vi "Obtain Queue.vi"(8 "error in (no error)":errorcluster, 10 "Queue Name":string) -> (0 "error out":errorcluster, 3 "queue out":refnum<queue>)   [LabVIEW 2019, in "Status.lvlib"]
doc: "Function to enqueue a Message in a Queue of other Module."
uses:
  Status.lvlib
  Queue Type.ctl
  State Name.ctl
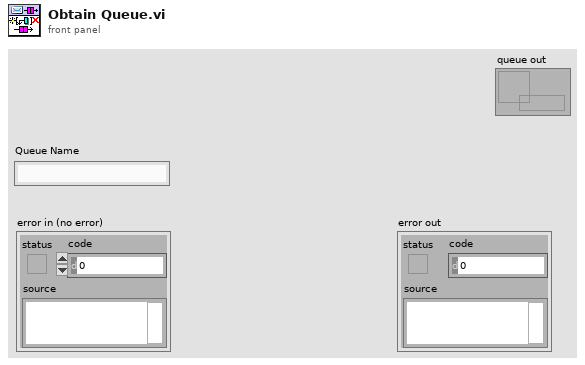
[diagram p1: front panel]
types:
  T1 = typedef "Status.lvlib/Queue Type.ctl" = cluster{"Custom State Name":string, "Defined State Name":T2, "Call Chain":string[], "Message Data":variant}
  T2 = typedef "Status.lvlib/State Name.ctl" = enum16{"Initialize", "Update Progress Bar", "Update Status Bar", "Set Cursor Busy", "Unset Cursor Busy", "Error", "Default", "Exit"}
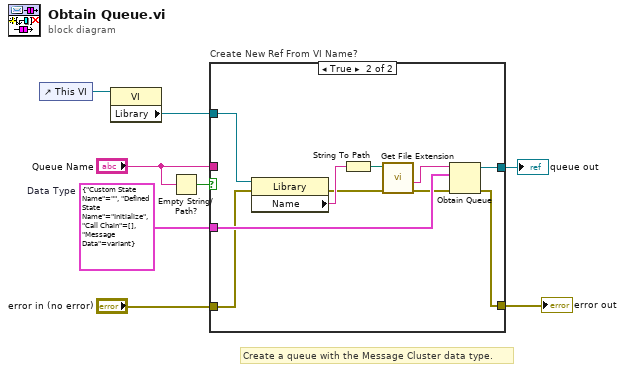
[diagram p0: block diagram]
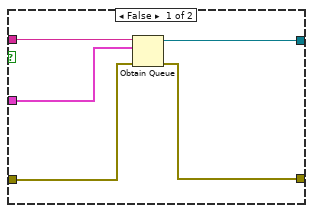
[diagram p2: hidden frame]
diagram:
  w6 = T1 {"Custom State Name"="", "Defined State Name"=enum."Initialize", "Call Chain"=[], "Message Data"=variant}  # Data Type
  # "Create a queue with the Message Cluster data type."
  n1 = control-ref of="This VI"() -> (w2:refnum<vi>)
  n2 = property class="VI"(reference=w2) -> ("Library"=w1:refnum<vi>)  [unwired: 1 in, 2 out]
  n3 = Empty String/Path?(string/path="Queue Name") -> (empty?=w8:bool)
  n4 = case "Create New Ref From VI Name?" shown="True" w8 {
    tunnel: "error in (no error)" -> [w13 w16]
    tunnel: [w12 w23] -> w5
    tunnel: [w11 w22] -> w3
    tunnel: "Queue Name" -> [w10 _]
    tunnel: w6 -> [w9 w21]
    tunnel: w1 -> [_ w20]
    frame False {
      n5 = Obtain Queue(name (unnamed)=w10, element data type=w9, error in (no error)=w13) -> (queue out=w11:refnum<queue>, error out=w12:errorcluster)  [unwired: 2 in, 1 out]
    }
    frame True {
      n6 = property class="Library"(reference=w20, error in=w16) -> (error out=w15:errorcluster, "Name"=w18:string)  [unwired: 1 out]
      n7 = String To Path(string=w18) -> (path=w17:path)
      n8 = call <vilib>:"Get File Extension.vi"("error in (no error)"=w15, "file"=w17) -> ("error out"=w14:errorcluster, "filename without extension"=w19:string)  [unwired: 8 out]
      n9 = Obtain Queue(name (unnamed)=w19, element data type=w21, error in (no error)=w14) -> (queue out=w22:refnum<queue>, error out=w23:errorcluster)  [unwired: 2 in, 1 out]
    }
  }
  "error out" <- w5
  "queue out" <- w3
